vi "Get Output.vi"(8 "error in (no error)":errorcluster, 11 "Keithley 2400 in":refnum<class "Keithley 2400.lvclass">) -> (0 "error out":errorcluster, 2 "output":bool, 3 "Keithley 2400 out":refnum<class "Keithley 2400.lvclass">)   [LabVIEW 2011, in "Keithley 2400.lvclass"]
uses:
  Keithley 2400.lvclass
  Keithley 2400.lvclass/Keithley 2400.ctl
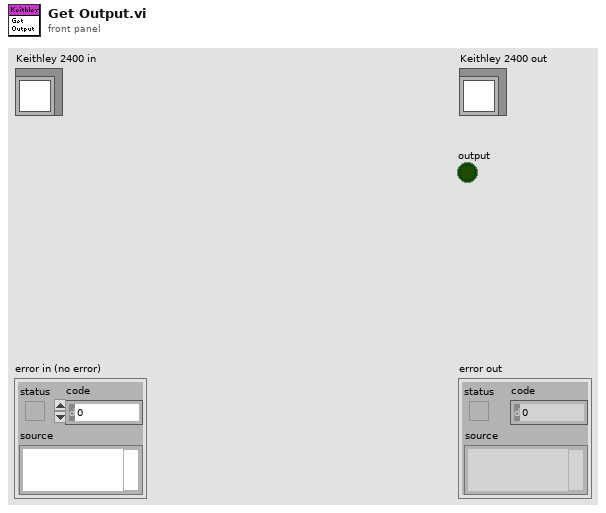
[diagram p1: front panel]
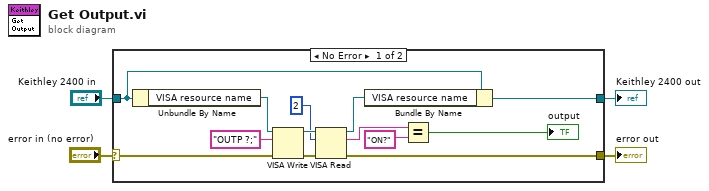
[diagram p0: block diagram]
diagram:
  n1 = case shown="No Error" "error in (no error)" {
    selector: "error in (no error)" -> [w14 w19]
    tunnel: [w12 w19] -> w3
    tunnel: [w8 w18] -> w1
    tunnel: "Keithley 2400 in" -> [w10 w18]
    frame No Error {
      n2 = Unbundle By Name(w10) -> ("VISA resource name"=w5:refnum<visa-resource-name>)
      n3 = VISA Write(VISA resource name=w5, write buffer="OUTP ?;", error in (no error)=w14) -> (VISA resource name out=w16:refnum<visa-resource-name>, error out=w13:errorcluster)  [unwired: 1 out]
      n4 = VISA Read(VISA resource name=w16, byte count=u32 2, error in (no error)=w13) -> (VISA resource name out=w9:refnum<visa-resource-name>, read buffer=w11:string, error out=w12:errorcluster)  [unwired: 1 out]
      n5 = Bundle By Name(cluster=w10, "VISA resource name"=w9) -> (w8:refnum<class "Keithley 2400.lvclass">)
      n6 = Equal?(x=w11, y="ON?") -> (x = y?=→"output":bool)
    }
    frame Error {
    }
  }
  "error out" <- w3
  "Keithley 2400 out" <- w1
